vi "Update-active-display.vi"(6 "Active display":T1, 8 "error in (no error)":errorcluster, 9 "Image refs":T2[](array[typedef]), 10 "Data ref. in":refnum<data-value>, 11 "UI ref. in":refnum<data-value>) -> (0 "error out":errorcluster, 2 "Data ref.":refnum<data-value>, 3 "UI ref.":refnum<data-value>)   [LabVIEW 2013, in "CameraVision.lvlib" / "CV-UI.lvclass"]
uses:
  CV-UI.lvclass
  <vilib>/vision/Image Controls.llb/IMAQ Image.ctl
  Main/CV-Main.lvclass
  Display-selector.ctl
  Display-names.ctl
  CV-UI.lvclass/CV-UI.ctl
  Read Camera.vi
  <vilib>/vision/NI_Vision_Development_Module.lvlib
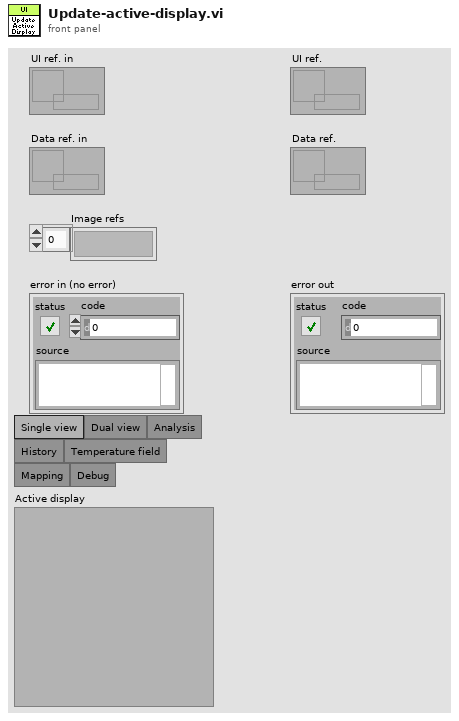
[diagram p1: front panel]
types:
  T1 = typedef "CameraVision.lvlib/CV-UI.lvclass/Display-selector.ctl" = enum32{"Single view", "Dual view", "Analysis", "History", "Temperature field", "Mapping", "Debug"}
  T2 = typedef "IMAQ Image.ctl" = refnum<image>
  T3 = typedef "CameraVision.lvlib/CV-UI.lvclass/Display-names.ctl" = enum16{"State", "Action", "Current image", "Framerate", "Frametime", "Process buffer", "Storage buffer", "Free disk space", "Total disk space", "Information", "Histogram", "Camera 1", "Camera 2", "Camera 1 chart", "Camera 2 chart", "Browser", "Temperature", "Map", "Status overview", "Characteristics", "Temper characteristics"}
  T4 = typedef "CameraVision.lvlib/CV-UI.lvclass/Camera-selector.ctl" = enum16{"Camera 1", "Camera 2"}
  T5 = typedef "CameraVision.lvlib/CV-Buffers.lvclass/Storage-buffer.ctl" = cluster{"Index":i32, "Time":timestamp, "Raw images":T2[], "Corrected images":T2[], "Binary images":T2[], "Temperature characteristics":T6, "Characteristics":T7[], "Temperature field":dbl[][]}
  T6 = typedef "CameraVision.lvlib/CV-Temperature.lvclass/Temperature-characteristics.ctl" = cluster{"Average temperature ":dbl, "Max. temperature":dbl, "Min. temperature":dbl, "Stand. dev. temperature":dbl, "Datapoints":dbl}
  T7 = typedef "CameraVision.lvlib/CV-Analysis.lvclass/Characteristics-cluster.ctl" = cluster{"Average intensity":dbl, "Peak intensity":dbl, "Melt-pool size":dbl, "Melt-pool aspect ratio":dbl, "Melt-pool fragments":dbl, "Centre of mass X":dbl, "Centre of mass Y":dbl, "Orientation":dbl}
  T8 = cluster{"Starting Value":sgl, "Incremental Value":sgl, "Histogram":u32[]}
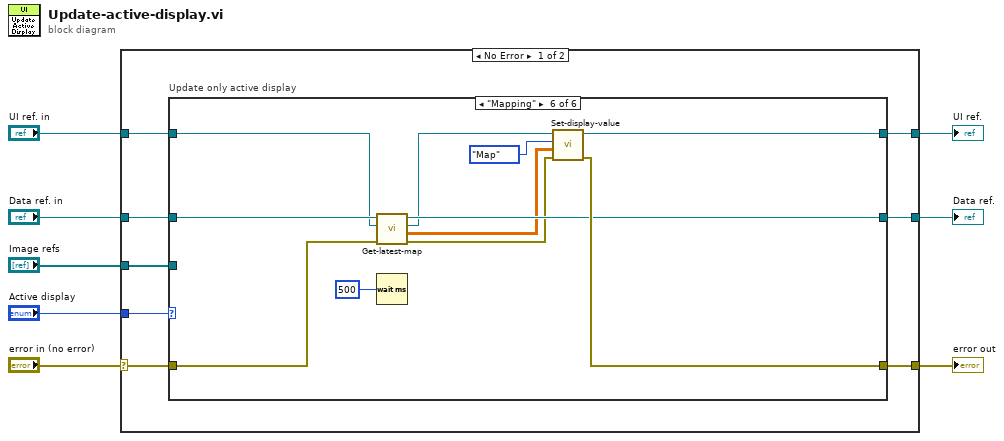
[diagram p0: block diagram]
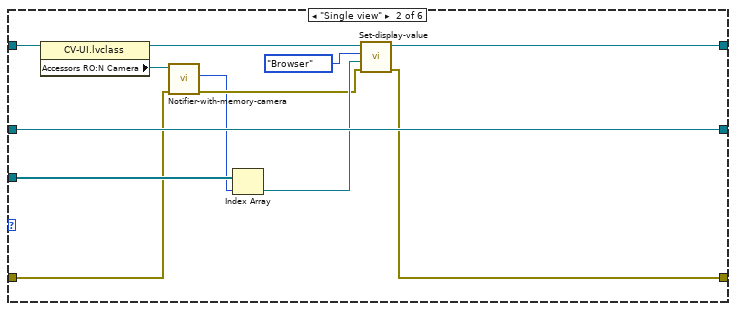
[diagram p3: hidden frame]
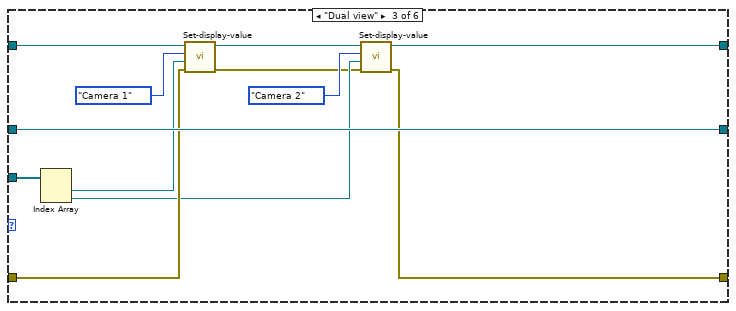
[diagram p4: hidden frame]
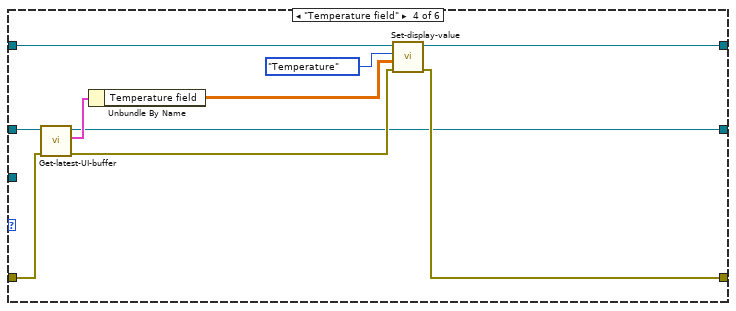
[diagram p5: hidden frame]
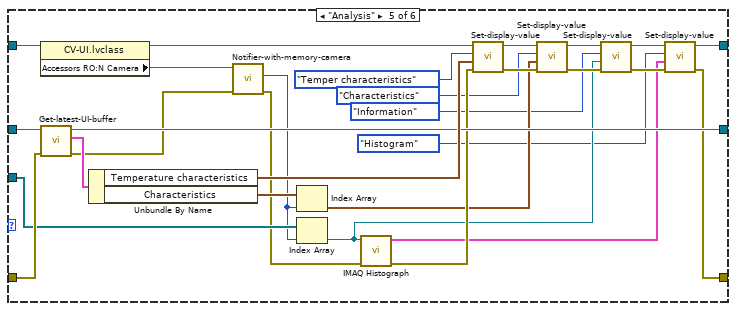
[diagram p6: hidden frame]
diagram:
  n1 = case shown="No Error" "error in (no error)" {
    selector: "error in (no error)" -> [w9 w94]
    tunnel: [w16 w96] -> w8
    tunnel: "Image refs" -> [w15 _]
    tunnel: "Data ref. in" -> [w14 w95]
    tunnel: [w13 w94] -> w5
    tunnel: [w12 w95] -> w4
    tunnel: "UI ref. in" -> [w11 w96]
    tunnel: "Active display" -> [w10 _]
    frame No Error {
      n2 = case "Update only active display" shown="\"Mapping\"" w10 {
        tunnel: w14 -> [w19 w31 w43 w50 w81 w91]
        tunnel: [w17 w22 w40 w45 w61 w89] -> w13
        tunnel: [w19 w31 w43 w44 w77 w88] -> w12
        tunnel: w9 -> [w17 w23 w37 w49 w80 w90]
        tunnel: w11 -> [w18 w30 w33 w51 w75 w86]
        tunnel: w15 -> [_ w28 w42 _ w73 _]
        tunnel: [w18 w21 w39 w52 w63 w92] -> w16
        frame Default {
        }
        frame "Single view" {
          n3 = property class="CV-UI.lvclass"(reference=w30) -> (reference out=w27:refnum<data-value>, "Accessors RO:N Camera"=w29:refnum<notifier>)  [unwired: 1 in, 1 out]
          n4 = call "Notifier-with-memory-camera.vi"("error in"=w23, "Notifier in"=w29) -> ("error IO"=w24:errorcluster, "Notification"=w20:T4)  [unwired: 8 in]
          n5 = Index Array(array=w28, index=w20) -> (element=w25:T2)
          n6 = call "Set-display-value.vi"("error in (no error)"=w24, "Value"=w25, "Display name"=Display-names."Browser", "UI ref. in"=w27) -> ("error out"=w22:errorcluster, "UI ref."=w21:refnum<data-value>)  [unwired: 6 in]
        }
        frame "Dual view" {
          n7 = Index Array(array=w42) -> (element #1=w36:T2, element #2=w35:T2)  [unwired: 2 in]
          n8 = call "Set-display-value.vi"("error in (no error)"=w37, "Value"=w36, "Display name"=Display-names."Camera 1", "UI ref. in"=w33) -> ("error out"=w34:errorcluster, "UI ref."=w32:refnum<data-value>)  [unwired: 6 in]
          n9 = call "Set-display-value.vi"("error in (no error)"=w34, "Value"=w35, "Display name"=Display-names."Camera 2", "UI ref. in"=w32) -> ("error out"=w40:errorcluster, "UI ref."=w39:refnum<data-value>)  [unwired: 6 in]
        }
        frame "Temperature field" {
          n10 = call "Get-latest-UI-buffer.vi"("error in (no error)"=w49, "Data ref. in"=w50) -> ("error out"=w46:errorcluster, "UI buffer"=w48:T5, "Data ref."=w44:refnum<data-value>)  [unwired: 7 in]
          n11 = Unbundle By Name(w48) -> ("Temperature field"=w47:dbl[][])
          n12 = call "Set-display-value.vi"("error in (no error)"=w46, "Value"=w47, "Display name"=Display-names."Temperature", "UI ref. in"=w51) -> ("error out"=w45:errorcluster, "UI ref."=w52:refnum<data-value>)  [unwired: 6 in]
        }
        frame "Analysis" {
          n13 = property class="CV-UI.lvclass"(reference=w75) -> (reference out=w70:refnum<data-value>, "Accessors RO:N Camera"=w76:refnum<notifier>)  [unwired: 1 in, 1 out]
          n14 = call "Get-latest-UI-buffer.vi"("error in (no error)"=w80, "Data ref. in"=w81) -> ("error out"=w71:errorcluster, "UI buffer"=w79:T5, "Data ref."=w77:refnum<data-value>)  [unwired: 7 in]
          n15 = Unbundle By Name(w79) -> ("Temperature characteristics"=w78:T6, "Characteristics"=w74:T7[])
          n16 = call "Notifier-with-memory-camera.vi"("error in"=w71, "Notifier in"=w76) -> ("error IO"=w60:errorcluster, "Notification"=w72:T4)  [unwired: 8 in]
          n17 = Index Array(array=w74, index=w72) -> (element=w58:T7)
          n18 = Index Array(array=w73, index=w72) -> (element=w56:T2)
          n19 = call "IMAQ Histograph"("error in (no error)"=w60, "Image"=w56) -> ("error out"=w62:errorcluster, "Histogram Graph"=w54:T8)  [unwired: 6 in, 2 out]
          n20 = call "Set-display-value.vi"("error in (no error)"=w62, "Value"=w78, "Display name"=Display-names."Temper characteristics", "UI ref. in"=w70) -> ("error out"=w69:errorcluster, "UI ref."=w68:refnum<data-value>)  [unwired: 6 in]
          n21 = call "Set-display-value.vi"("error in (no error)"=w69, "Value"=w58, "Display name"=Display-names."Characteristics", "UI ref. in"=w68) -> ("error out"=w67:errorcluster, "UI ref."=w66:refnum<data-value>)  [unwired: 6 in]
          n22 = call "Set-display-value.vi"("error in (no error)"=w67, "Value"=w56, "Display name"=Display-names."Information", "UI ref. in"=w66) -> ("error out"=w65:errorcluster, "UI ref."=w64:refnum<data-value>)  [unwired: 6 in]
          n23 = call "Set-display-value.vi"("error in (no error)"=w65, "Value"=w54, "Display name"=Display-names."Histogram", "UI ref. in"=w64) -> ("error out"=w61:errorcluster, "UI ref."=w63:refnum<data-value>)  [unwired: 6 in]
        }
        frame "Mapping" {
          n24 = call "Get-latest-map.vi"("error in (no error)"=w90, "UI ref. in"=w86, "Data ref. in"=w91) -> ("error out"=w84:errorcluster, "2D map"=w83:dbl[][], "UI ref."=w85:refnum<data-value>, "Data ref."=w88:refnum<data-value>)  [unwired: 5 in]
          n25 = Wait (ms)(milliseconds to wait=u32 500) -> ()  [unwired: 1 out]
          n26 = call "Set-display-value.vi"("error in (no error)"=w84, "Value"=w83, "Display name"=Display-names."Map", "UI ref. in"=w85) -> ("error out"=w89:errorcluster, "UI ref."=w92:refnum<data-value>)  [unwired: 6 in]
        }
      }
    }
    frame Error {
    }
  }
  "UI ref." <- w8
  "error out" <- w5
  "Data ref." <- w4
